vi "GetDeviceStatus.vi"(8 "error in (no error)":errorcluster, 11 "Camera_Prime95B in":refnum<class "Camera_Prime95B.lvclass">) -> (0 "error out":errorcluster, 2 "Status":T1 items=["Idle", "Busy"], 3 "Camera_Prime95B out":refnum<class "Camera_Prime95B.lvclass">)   [LabVIEW 2020, in "Camera_Prime95B.lvlib" / "Camera_Prime95B.lvclass"]
uses:
  Camera_Prime95B.lvclass
  Hardware Abstraction Layer/Component/Device/Device/DeviceStatus.ctl
  Camera_Prime95B.lvclass/Camera_Prime95B.ctl
  E:/Development/DevHardSoftware/MicroscopyFramework/Model/Hardware Layer/Real Hardware/Camera_Prime95B/Camera_Prime95B/Dependencies/PVCamNET.dll
  Dependencies/PVCamNET.dll
  Hardware Abstraction Layer/Component/Camera/Camera/Camera.lvclass
  Hardware Abstraction Layer/Component/Device/Device.lvlib
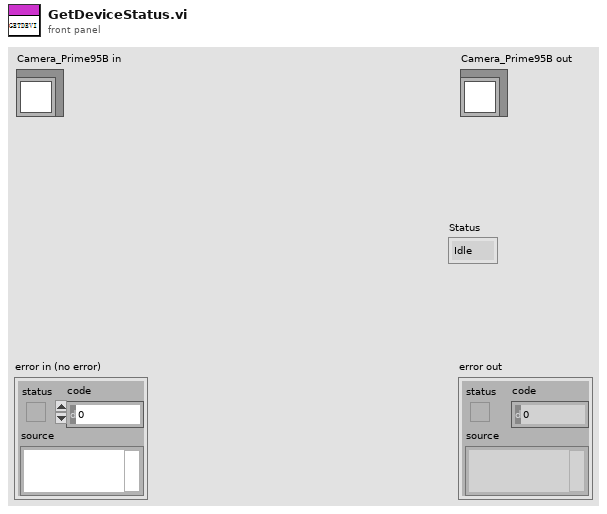
[diagram p1: front panel]
types:
  T1 = typedef "Device.lvlib/DeviceStatus.ctl" = i32
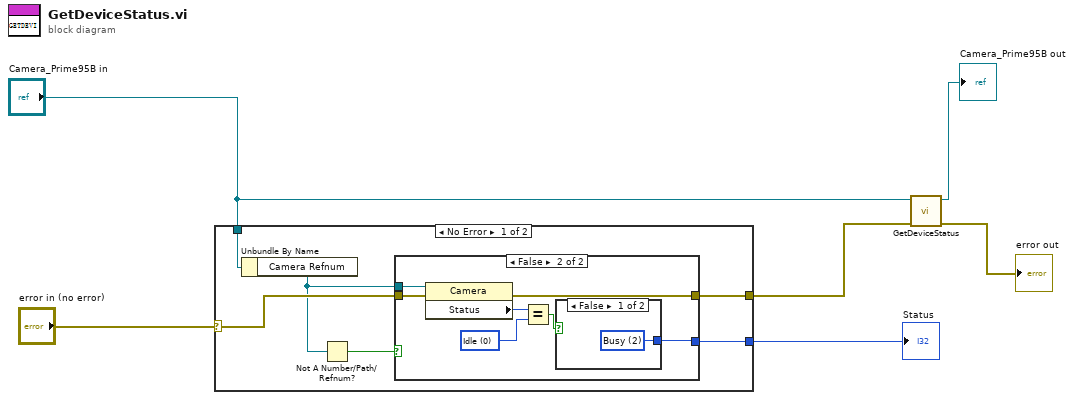
[diagram p0: block diagram]
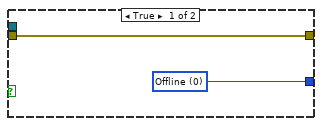
[diagram p2: hidden frame]
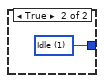
[diagram p3: hidden frame]
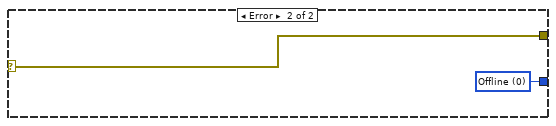
[diagram p4: hidden frame]
diagram:
  n1 = case shown="No Error" "error in (no error)" {
    selector: "error in (no error)" -> [w10 w25]
    tunnel: [w11 w25] -> w2
    tunnel: "Camera_Prime95B in" -> [w12 _]
    tunnel: [w7 w24] -> w1
    frame No Error {
      n2 = Unbundle By Name(w12) -> ("Camera Refnum"=w9:refnum<k24>)
      n3 = Not A Number/Path/Refnum?(number/path/refnum=w9) -> (NaN/Path/Refnum?=w8:bool)
      n4 = case shown="False" w8 {
        tunnel: w9 -> [_ w21]
        tunnel: [w14 w20] -> w11
        tunnel: w10 -> [w14 w19]
        tunnel: [w13 w15] -> w7
        frame True {
          w13 = T1 0 items=["Offline", "Idle", "Busy"] ("Status")
        }
        frame False {
          w17 = 0 items=["Idle", "Capturing"] ("Status")
          n5 = property class="Camera"(reference=w21, error in=w19) -> (error out=w20:errorcluster, "Status"=w18:i32)  [unwired: 1 out]
          n6 = Equal?(x=w18, y=w17) -> (x = y?=w16:bool)
          n7 = case shown="False" w16 {
            tunnel: [w22 w23] -> w15
            frame False {
              w22 = T1 2 items=["Offline", "Idle", "Busy"] ("Status")
            }
            frame True {
              w23 = T1 1 items=["Offline", "Idle", "Busy"] ("Status")
            }
          }
        }
      }
    }
    frame Error {
      w24 = T1 0 items=["Offline", "Idle", "Busy"] ("Status")
    }
  }
  "Status" <- w1
  n8 = call-parent "GetDeviceStatus.vi"("error in (no error)"=w2, "Device in"="Camera_Prime95B in") -> ("error out"=→"error out":errorcluster, "Device out"=→"Camera_Prime95B out":refnum<class "Camera_Prime95B.lvclass">)  [unwired: 7 in, 1 out]
